vi "SCCSup FuncSupportedFromSuppCaps.vi"(2 "functionality":T1, 7 "suppCaps bit array":bool[](array[boolean])) -> (8 "functionality supported?":bool)   [LabVIEW 2020]
uses:
  <vilib>/SourceControl/sccapi/SCCAPI SCC Provider Functionality.ctl
  <vilib>/SourceControl/sccapi/NI_SCC.lvlib
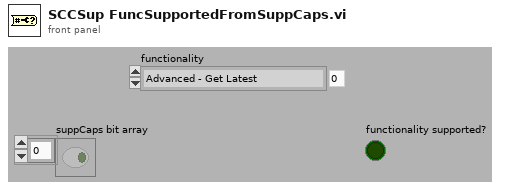
[diagram p1: front panel]
types:
  T1 = typedef "NI_SCC.lvlib/SCCAPI SCC Provider Functionality.ctl" = enum16{"Advanced - Get Latest", "Advanced - CheckOut", "Advanced - CheckIn", "Advanced - UndoCheckOut", "Advanced - Add", "Advanced - Remove", "Advanced - FileCompare", "Advanced - FileHistory", "Advanced - FileProperties", "Advanced - ConfigOptions", "Run SCC", "Configure Project", "Comment on CheckOut", "Comment on CheckIn", "Comment on Add", "Comment on Remove", "Keep Checked Out", "Get File Copy", "Multifile History"}
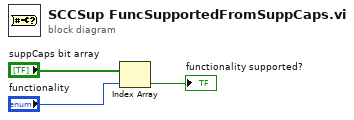
[diagram p0: block diagram]
diagram:
  n1 = Index Array(array="suppCaps bit array", index="functionality") -> (element=→"functionality supported?":bool)
